vi "GUI.DAQmxName.Set.vi"(8 "error in (no error)":errorcluster, 10 "deviceDAQConnect":tag, 11 "deviceDAQName":string) -> (0 "error out":errorcluster)   [LabVIEW 2019]
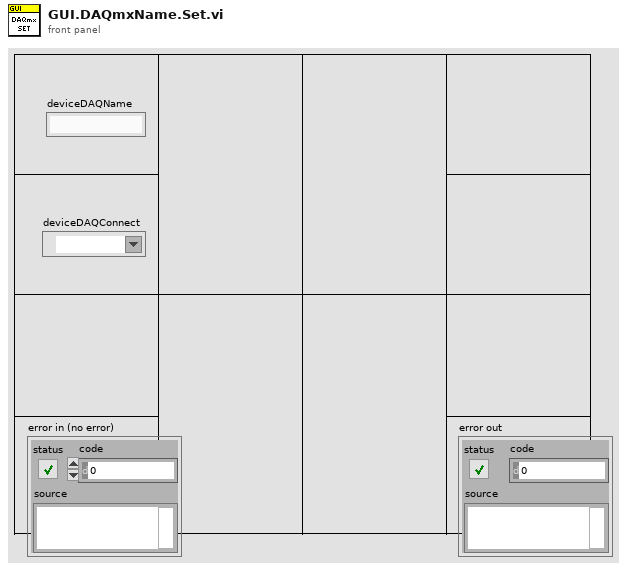
[diagram p1: front panel]
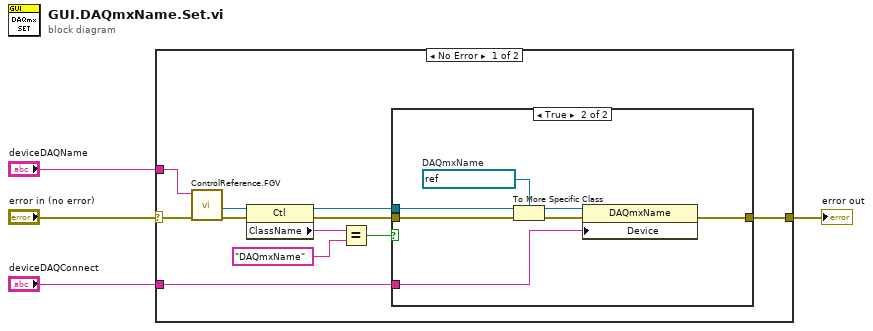
[diagram p0: block diagram]
diagram:
  n1 = case shown="No Error" "error in (no error)" {
    selector: "error in (no error)" -> [w15 w24]
    tunnel: [w9 w24] -> w2
    tunnel: "deviceDAQName" -> [w14 _]
    tunnel: "deviceDAQConnect" -> [w5 _]
    frame No Error {
      n2 = call "ControlReference.FGV.vi"("error in (no error)"=w15, "controlLabelText"=w14) -> ("error out"=w13:errorcluster, "referenceToControl"=w12:refnum<vi>)  [unwired: 8 in]
      n3 = property class="Ctl"(reference=w12, error in=w13) -> (reference out=w8:refnum<vi>, error out=w10:errorcluster, "ClassName"=w11:string)
      n4 = Equal?(x=w11, y="DAQmxName") -> (x = y?=w7:bool)
      n5 = case shown="True" w7 {
        tunnel: w10 -> [w16 w23]
        tunnel: [w16 w18] -> w9
        tunnel: w8 -> [_ w22]
        tunnel: w5 -> [_ w17]
        frame False {
        }
        frame True {
          w21 = refnum<vi> refnum  # DAQmxName
          n6 = To More Specific Class(target class=w21, reference=w22, error in=w23) -> (specific class reference=w20:refnum<vi>, error out=w19:errorcluster)
          n7 = property class="DAQmxName"(reference=w20, error in=w19, "Device"=w17) -> (error out=w18:errorcluster)  [unwired: 1 out]
        }
      }
    }
    frame Error {
    }
  }
  "error out" <- w2
